vi "GetCrosshairVector.vi"(8 "Target Crosshair":string(combo), 11 "Current Crosshair":string(combo)) -> (2 "XY Vector":dbl[](array[numeric]))   [LabVIEW 2015]
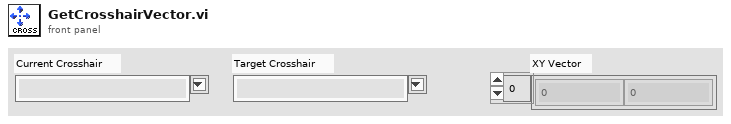
[diagram p1: front panel]
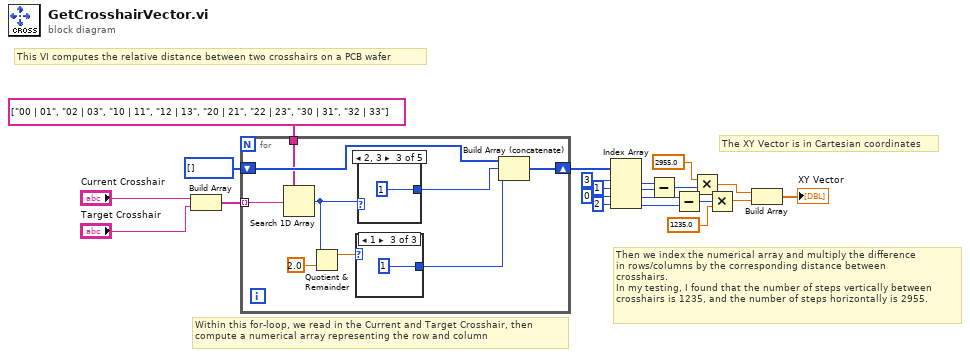
[diagram p0: block diagram]
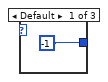
[diagram p2: hidden frame]
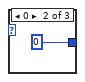
[diagram p3: hidden frame]
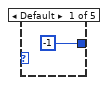
[diagram p4: hidden frame]
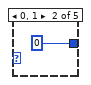
[diagram p5: hidden frame]
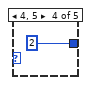
[diagram p6: hidden frame]
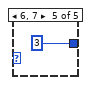
[diagram p7: hidden frame]
diagram:
  # "Then we index the numerical array and multiply the difference\nin rows/columns by the corresponding distance between\ncrosshairs.\nIn my testing, I found that the number of steps vertically between\ncrosshairs is 1235, and the number of steps horizontally is 2955."
  # "Within this for-loop, we read in the Current and Target Crosshair, then \ncompute a numerical array representing the row and column"
  # "The XY Vector is in Cartesian coordinates"
  # "This VI computes the relative distance between two crosshairs on a PCB wafer"
  n1 = Build Array("Current Crosshair", "Target Crosshair") -> (w18:string[])
  n2 = for {
    tunnel: string[] ["00 | 01", "02 | 03", "10 | 11", "12 | 13", "20 | 21", "22 | 23", "30 | 31", "32 | 33"] -> [w24]
    tunnel: w18 -> [w23] mode=indexing
    shift-right: [w26] -> w16
    shift-left: i32[] [] -> [w25]
    n3 = Search 1D Array(1D array=w24, element=w23) -> (index of element=w22:i32)  [unwired: 1 in]
    n4 = Quotient & Remainder(x=w22, y=2.0) -> (x-y*floor(x/y)=w29:dbl)  [unwired: 1 out]
    n5 = case shown="1" w29 {
      tunnel: [-1 0 1] -> w27
      frame Default {
      }
      frame 0 {
      }
      frame 1 {
      }
    }
    n6 = case shown="2, 3" w22 {
      tunnel: [-1 0 1 2 3] -> w28
      frame Default {
      }
      frame 0, 1 {
      }
      frame 2, 3 {
      }
      frame 4, 5 {
      }
      frame 6, 7 {
      }
    }
    n7 = Build Array (concatenate)(w25, w28, w27) -> (w26:i32[])
  }
  n8 = Index Array(array=w16, index #1=3 ("index"), index #2=1 ("index"), index #3=0 ("index"), index #4=2 ("index")) -> (element #1=w9:i32, element #2=w8:i32, element #3=w11:i32, element #4=w10:i32)
  n9 = Subtract(x=w9, y=w8) -> (x-y=w5:i32)
  n10 = Subtract(x=w11, y=w10) -> (x-y=w4:i32)
  n11 = Multiply(x=2955.0, y=w5) -> (x*y=w3:dbl)
  n12 = Multiply(x=w4, y=1235.0) -> (x*y=w2:dbl)
  n13 = Build Array(w3, w2) -> (→"XY Vector":dbl[])
